vi "FinalizeHWI.vi"(8 "error in (no error)":errorcluster, 10 "Master Device in":refnum<class "Master Device.lvclass">, 11 "DDS in":refnum<class "DDS.lvclass">) -> (0 "error out":errorcluster, 2 "Master Device out":refnum<class "Master Device.lvclass">, 3 "DDS out":refnum<class "DDS.lvclass">)   [LabVIEW 2013, in "DDS.lvclass"]
uses:
  DDS.lvclass
  Master Device/Master Device.lvclass
  DDS.lvclass/DDS.ctl
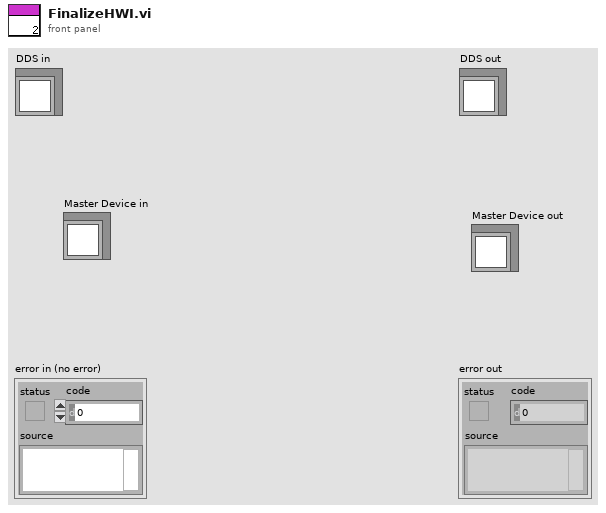
[diagram p1: front panel]
types:
  T1 = typedef "SlaveInfo.ctl" = cluster{"Triggering":bool[][], "Ramp Info":T2[]}
  T2 = typedef "RampInfo.ctl" = cluster{"Table Ramp Index":i32, "Ramp Time":dbl, "Number of Steps":i32, "Instruction Array Index":i32}
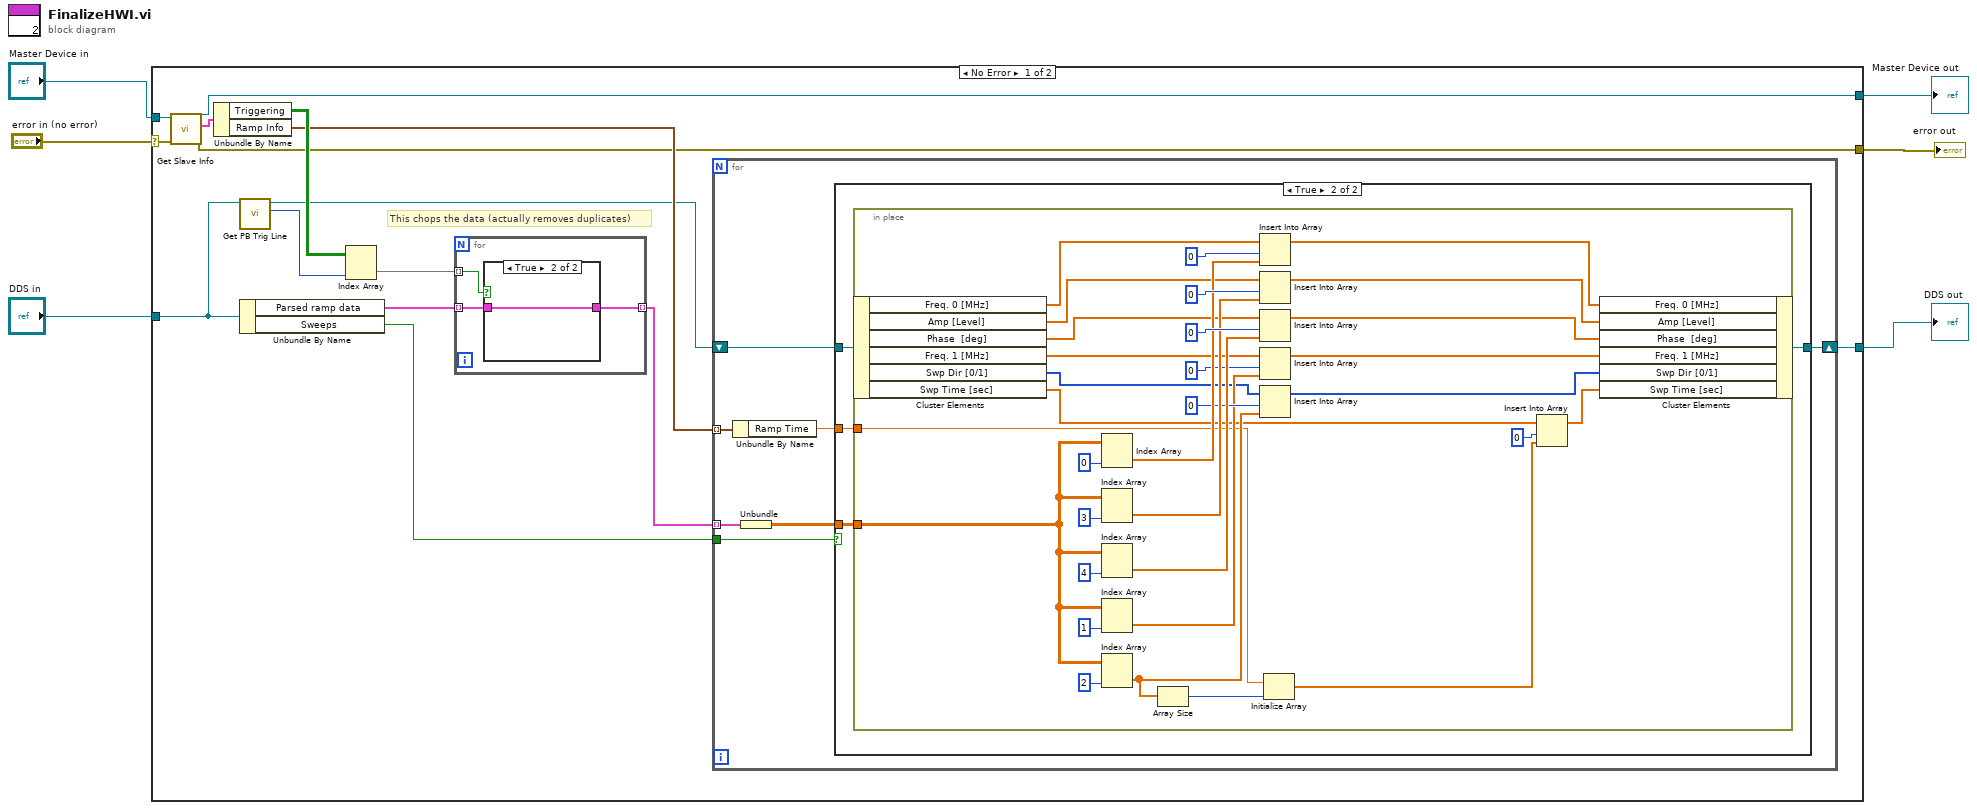
[diagram p0: block diagram]
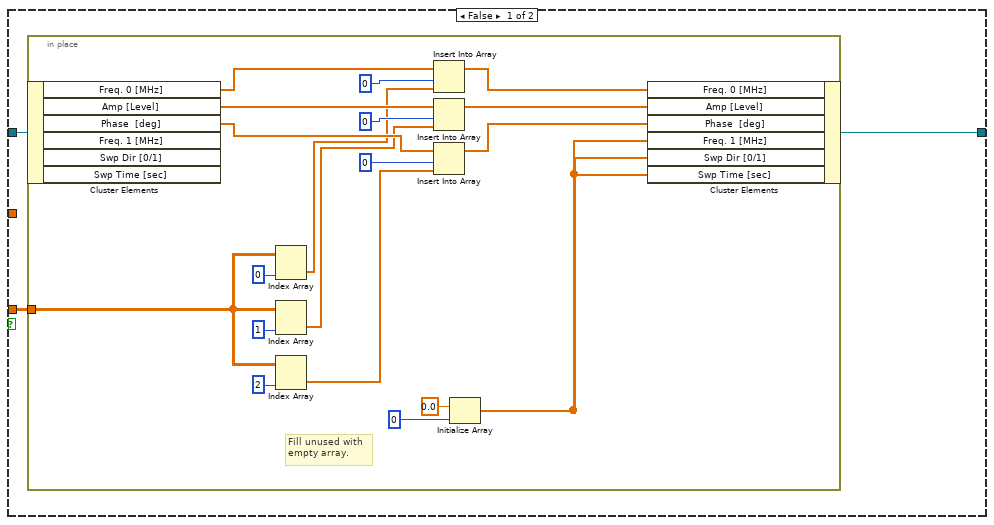
[diagram p2: hidden frame]
diagram:
  n1 = case shown="No Error" "error in (no error)" {
    selector: "error in (no error)" -> [w17 w93]
    tunnel: [w7 w93] -> w5
    tunnel: "Master Device in" -> [w18 w92]
    tunnel: "DDS in" -> [w16 w91]
    tunnel: [w8 w91] -> w2
    tunnel: [w13 w92] -> w1
    frame No Error {
      # "This chops the data (actually removes duplicates)"
      n2 = call-dynamic "Get Slave Info.vi"("error in (no error)"=w17, "Master Device in"=w18) -> ("error out"=w7:errorcluster, "Slave Info"=w21:T1, "Master Device out"=w13:refnum<class "Master Device.lvclass">)  [unwired: 7 in]
      n3 = Unbundle By Name(w21) -> ("Triggering"=w20:bool[][], "Ramp Info"=w11:T2[])
      n4 = call-dynamic "Get PB Trig Line.vi"("Device in"=w16) -> ("PB Trigger Line"=w19:u16, "Device out"=w9:refnum<class "DDS.lvclass">)  [unwired: 8 in, 1 out]
      n5 = Unbundle By Name(w16) -> ("Parsed ramp data"=w15:cluster{"Ramp Element":dbl[][]}[], "Sweeps"=w12:bool)
      n6 = Index Array(array=w20, index (col)=w19) -> (element=w14:bool[])  [unwired: 1 in]
      n7 = for {
        tunnel: w15 -> [w89] mode=indexing
        tunnel: [w87] -> w10 mode=indexing
        tunnel: w14 -> [w88] mode=indexing
        n8 = case shown="True" w88 {
          tunnel: [_ w90] -> w87
          tunnel: w89 -> [_ w90]
          frame False {
          }
          frame True {
          }
        }
      }
      n9 = for {
        tunnel: w10 -> [w23] mode=indexing
        tunnel: w12 -> [w26]
        shift-right: [w28] -> w8
        shift-left: w9 -> [w27]
        tunnel: w11 -> [w24] mode=indexing
        n10 = Unbundle By Name(w24) -> ("Ramp Time"=w25:dbl)
        n11 = Unbundle(w23) -> ("Ramp Element"=w22:dbl[][])
        n12 = case shown="True" w26 {
          tunnel: w22 -> [w29 w52]
          tunnel: [w30 w53] -> w28
          tunnel: w27 -> [w31 w54]
          tunnel: w25 -> [_ w51]
          frame False {
            n13 = in-place {
              in-place-border: w29 -> [w32]
              # "Fill unused with\nempty array."
              n14 = in-place-cluster #1(w31) -> ("Freq. 0 [MHz]"=w44:dbl[], "Amp [Level]"=w43:dbl[], "Phase  [deg]"=w42:dbl[])  [unwired: 3 out]
              n15 = Index Array(array=w32, index (col)=0 ("disabled index (col)")) -> (element=w41:dbl[])  [unwired: 1 in]
              n16 = Index Array(array=w32, index (col)=1 ("disabled index (col)")) -> (element=w40:dbl[])  [unwired: 1 in]
              n17 = Index Array(array=w32, index (col)=2 ("disabled index (col)")) -> (element=w39:dbl[])  [unwired: 1 in]
              n18 = Insert Into Array(array=w44, index=0, new element=w41) -> (w38:dbl[])
              n19 = Insert Into Array(array=w43, index=0, new element=w40) -> (w37:dbl[])
              n20 = Insert Into Array(array=w42, index=0, new element=w39) -> (w36:dbl[])
              n21 = Initialize Array(0.0 ("element"), 0 ("dimension size")) -> (w33:dbl[])
              n22 = in-place-cluster #1("Freq. 0 [MHz]"=w38, "Amp [Level]"=w37, "Phase  [deg]"=w36, "Freq. 1 [MHz]"=w33, "Swp Dir [0/1]"=w33, "Swp Time [sec]"=w33) -> (w30:refnum<class "DDS.lvclass">)
            }
          }
          frame True {
            n23 = in-place {
              in-place-border: w52 -> [w55]
              in-place-border: w51 -> [w57]
              n24 = in-place-cluster #2(w54) -> ("Freq. 0 [MHz]"=w78:dbl[], "Amp [Level]"=w74:dbl[], "Phase  [deg]"=w72:dbl[], "Freq. 1 [MHz]"=w66:dbl[], "Swp Dir [0/1]"=w63:i32[], "Swp Time [sec]"=w59:dbl[])
              n25 = Index Array(array=w55, index (col)=0 ("disabled index (col)")) -> (element=w77:dbl[])  [unwired: 1 in]
              n26 = Index Array(array=w55, index (col)=3 ("disabled index (col)")) -> (element=w75:dbl[])  [unwired: 1 in]
              n27 = Index Array(array=w55, index (col)=4 ("disabled index (col)")) -> (element=w70:dbl[])  [unwired: 1 in]
              n28 = Index Array(array=w55, index (col)=1 ("disabled index (col)")) -> (element=w64:dbl[])  [unwired: 1 in]
              n29 = Index Array(array=w55, index (col)=2 ("disabled index (col)")) -> (element=w61:dbl[])  [unwired: 1 in]
              n30 = Array Size(array=w61) -> (size(s)=w60:i32)
              n31 = Insert Into Array(array=w78, index=0, new element=w77) -> (w76:dbl[])
              n32 = Insert Into Array(array=w74, index=0, new element=w75) -> (w73:dbl[])
              n33 = Insert Into Array(array=w72, index=0, new element=w70) -> (w71:dbl[])
              n34 = Insert Into Array(array=w66, index=0, new element=w64) -> (w65:dbl[])
              n35 = Insert Into Array(array=w63, index=0, new element=w61) -> (w62:i32[])
              n36 = Initialize Array(w57, w60) -> (w56:dbl[])
              n37 = Insert Into Array(array=w59, index=0, new element=w56) -> (w58:dbl[])
              n38 = in-place-cluster #2("Freq. 0 [MHz]"=w76, "Amp [Level]"=w73, "Phase  [deg]"=w71, "Freq. 1 [MHz]"=w65, "Swp Dir [0/1]"=w62, "Swp Time [sec]"=w58) -> (w53:refnum<class "DDS.lvclass">)
            }
          }
        }
      }
    }
    frame Error {
    }
  }
  "error out" <- w5
  "DDS out" <- w2
  "Master Device out" <- w1
